vi "WDT Waveform Duration DBL.vi"(7 "open interval? (T)":bool=TRUE, 8 "error in (no error)":errorcluster, 11 "waveform in":waveform(dbl)) -> (0 "error out":errorcluster, 2 "duration":dbl format="%0.2f", 3 "waveform out":waveform(dbl))   [LabVIEW 2020]
doc: "Computes the <B>duration</B> of <B>waveform in</B> using the following equation: <B>duration</B> = (#samples-1) x dx. Wire data to the <B>waveform in</B> input to determine the polymorphic instance to use or manually select the instance."
panel:
  in  "Waveform ERROR":waveform(dbl)={"t0"=timestamp(0 s since 1904-01-01), "dt"=0.0, "Y"=[]}
  # "open"
  # "closed"
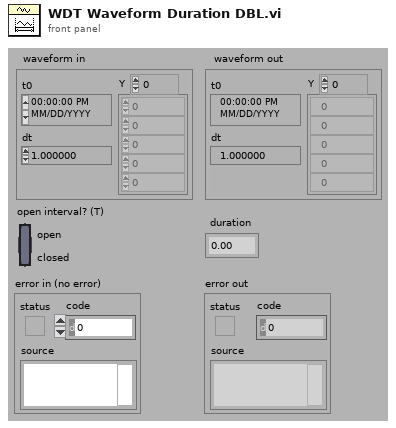
[diagram p1: front panel]
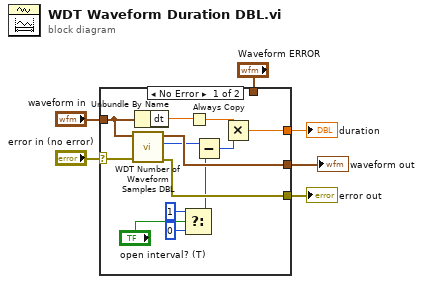
[diagram p0: block diagram]
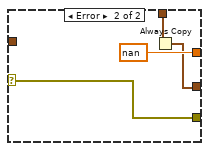
[diagram p2: hidden frame]
diagram:
  n1 = case shown="No Error" "error in (no error)" {
    selector: "error in (no error)" -> [w17 w21]
    tunnel: "waveform in" -> [w14 _]
    tunnel: [w16 nan] -> w6
    tunnel: [w13 w20] -> w5
    tunnel: "Waveform ERROR" -> [_ w22]
    tunnel: [w15 w21] -> w2
    frame No Error {
      n2 = call "WDT Number of Waveform Samples DBL.vi"("error in (no error)"=w17, "waveform in"=w14) -> ("error out"=w15:errorcluster, "number of samples"=w12:i32, "waveform out"=w13:waveform(dbl))  [unwired: 7 in]
      n3 = Unbundle By Name(w14) -> ("dt"=w19:dbl)
      n4 = Select(t=1 ("number of samples"), s="open interval? (T)", f=0 ("number of samples")) -> (s? t:f=w11:i32)
      n5 = Always Copy(1:w19) -> (0:w7:dbl)
      n6 = Subtract(x=w12, y=w11) -> (x-y=w18:i32)
      n7 = Multiply(x=w7, y=w18) -> (x*y=w16:dbl)
    }
    frame Error {
      # "Incoming Error"
      n8 = Always Copy(1:w22) -> (0:w20:waveform(dbl))
    }
  }
  "duration" <- w6
  "waveform out" <- w5
  "error out" <- w2
